vi "Patch data preview-Calculate TDMS data position.vi"(10 "Global cycle number among all trials":i32, 11 "Register cluster":T1) -> (1 "Cycle's data length":i64, 3 "Cycle's data start index in current trial":i64)   [LabVIEW 2020]
uses:
  Typedefs/Patch viewer internal cluster.ctl
  <vilib>/vision/Image Controls.llb/IMAQ Image.ctl
panel:
  out "Cycle index in current trial":i32
  out "Trial index":i32
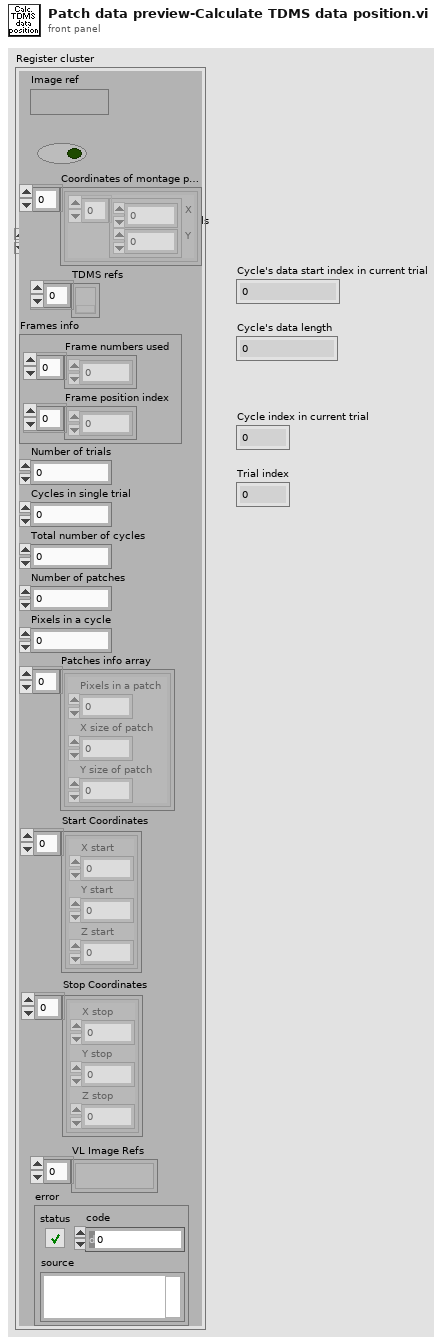
[diagram p1: front panel]
types:
  T1 = typedef "Patch viewer internal cluster.ctl" = cluster{"Image ref":T2, "Variable Length ?":bool, "Coordinates of montage positions":cluster{"X\n\nY":i32[]}[], "TDMS refs":refnum<k34>[], "Frames info":cluster{"Frame numbers used":i32[], "Frame position index":i32[]}, "Number of trials":i32, "Cycles in single trial":i32, "Total number of cycles":i32, "Number of patches":i32, "Pixels in a cycle":i32, "Patches info array":cluster{"Pixels in a patch":i32, "X size of patch":i32, "Y size of patch":i32}[], "Start Coordinates":cluster{"X start":i32, "Y start":i32, "Z start":i32}[], "Stop Coordinates":cluster{"X stop":i32, "Y stop":i32, "Z stop":i32}[], "VL Image Refs":T2[], "error":errorcluster}
  T2 = typedef "IMAQ Image.ctl" = refnum<image>
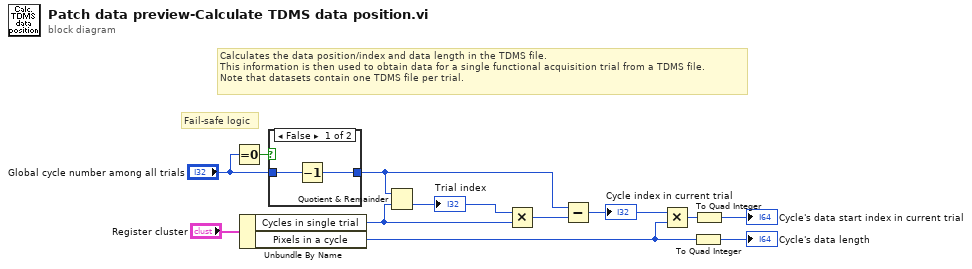
[diagram p0: block diagram]
diagram:
  # "Fail-safe logic"
  # "Calculates the data position/index and data length in the TDMS file.\nThis information is then used to obtain data for a single functional acquisition trial from a TDMS file.\nNote that datasets contain one TDMS file per trial."
  n1 = Equal To 0?(x="Global cycle number among all trials") -> (x = 0?=w2:bool)
  n2 = Unbundle By Name("Register cluster") -> ("Cycles in single trial"=w10:i32, "Pixels in a cycle"=w3:i32)
  n3 = case shown="False" w2 {
    tunnel: [w14 w15] -> w12
    tunnel: "Global cycle number among all trials" -> [w13 w15]
    frame False {
      n4 = Decrement(x=w13) -> (x-1=w14:i32)
    }
    frame True {
    }
  }
  n5 = Quotient & Remainder(x=w12, y=w10) -> (floor(x/y)=w9:i32)  [unwired: 1 out]
  "Trial index" <- w9
  n6 = Multiply(x=w9, y=w10) -> (x*y=w11:i32)
  n7 = Subtract(x=w12, y=w11) -> (x-y=w4:i32)
  "Cycle index in current trial" <- w4
  n8 = Multiply(x=w4, y=w3) -> (x*y=w5:i32)
  n9 = To Quad Integer(1:w3) -> (0:→"Cycle's data length":i64)
  n10 = To Quad Integer(1:w5) -> (0:→"Cycle's data start index in current trial":i64)
